vi "Xnet to Channel DT.vi"(10 "NumBits":u32, 11 "DataType":u32) -> (3 "data type":T1)   [LabVIEW 2013, in "J1939 configuration.lvclass"]
uses:
  J1939 configuration.lvclass
  <vilib>/NI/Tag Bus/tag/Data Type.ctl
  <vilib>/NI/Tag Bus/tag/tag descriptor.lvclass
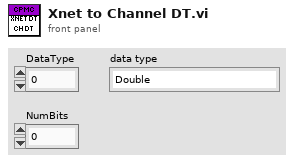
[diagram p1: front panel]
types:
  T1 = typedef "tag bus.lvlib/tag descriptor.lvclass/Data Type.ctl" = enum16{"Double", "Single", "I64", "I32", "I16", "I8", "U64", "U32", "U16", "U8", "Boolean", "String", "Array of Double", "Array of Single", "Array of I64", "Array of I32", "Array of I16", "Array of I8", "Array of U64", "Array of U32", "Array of U16", "Array of U8", "Array of Boolean", "Array of String"}
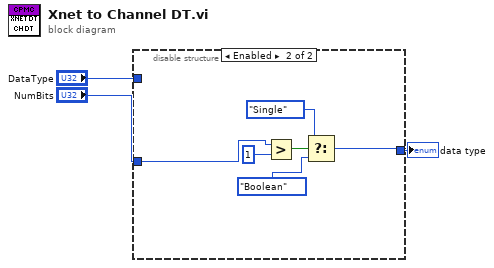
[diagram p0: block diagram]
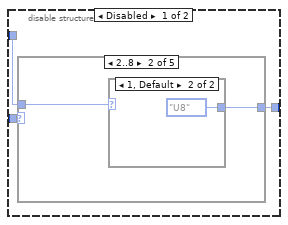
[diagram p2: hidden frame]
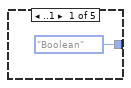
[diagram p3: hidden frame]
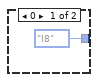
[diagram p4: hidden frame]
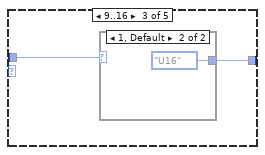
[diagram p5: hidden frame]
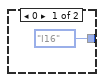
[diagram p6: hidden frame]
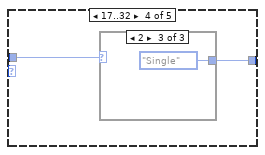
[diagram p7: hidden frame]
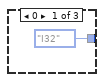
[diagram p8: hidden frame]
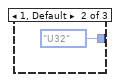
[diagram p9: hidden frame]
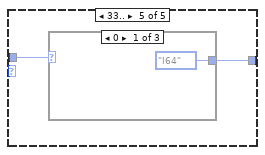
[diagram p10: hidden frame]
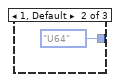
[diagram p11: hidden frame]
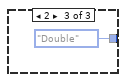
[diagram p12: hidden frame]
diagram:
  n1 = disable-structure shown="Enabled" {
    disable-tunnel: "DataType" -> [w6 _]
    disable-tunnel: "NumBits" -> [w5 w27]
    disable-tunnel: [w4 w26] -> w1
    frame Disabled {
      n2 = case shown="2..8" w5 {
        tunnel: [Data_Type."Boolean" ("data type") w9 w13 w17 w22] -> w4
        tunnel: w6 -> [_ w8 w12 w16 w21]
        frame ..1 {
        }
        frame 2..8 {
          n3 = case shown="1, Default" w8 {
            tunnel: [Data_Type."I8" ("data type") Data_Type."U8" ("data type")] -> w9
            frame 0 {
            }
            frame 1, Default {
            }
          }
        }
        frame 9..16 {
          n4 = case shown="1, Default" w12 {
            tunnel: [Data_Type."I16" ("data type") Data_Type."U16" ("data type")] -> w13
            frame 0 {
            }
            frame 1, Default {
            }
          }
        }
        frame 17..32 {
          n5 = case shown="2" w16 {
            tunnel: [Data_Type."I32" ("data type") Data_Type."U32" ("data type") Data_Type."Single" ("data type")] -> w17
            frame 0 {
            }
            frame 1, Default {
            }
            frame 2 {
            }
          }
        }
        frame 33.. {
          n6 = case shown="0" w21 {
            tunnel: [Data_Type."I64" ("data type") Data_Type."U64" ("data type") Data_Type."Double" ("data type")] -> w22
            frame 0 {
            }
            frame 1, Default {
            }
            frame 2 {
            }
          }
        }
      }
    }
    frame Enabled {
      n7 = Greater?(x=w27, y=u32 1) -> (0:w30:bool)
      n8 = Select(t=Data_Type."Single" ("data type"), s=w30, f=Data_Type."Boolean" ("data type")) -> (s? t:f=w26:T1)
    }
  }
  "data type" <- w1
